vi "clusterParsing.vi"() -> ()   [LabVIEW 2009]
uses:
  Publisher/dataCluster.ctl
  <vilib>/vision/Image Controls.llb/IMAQ Image.ctl
panel:
  out "Array":string[](array[string])
  in  "Cluster in 2":T1
  in  "Data cluster StateM":T3
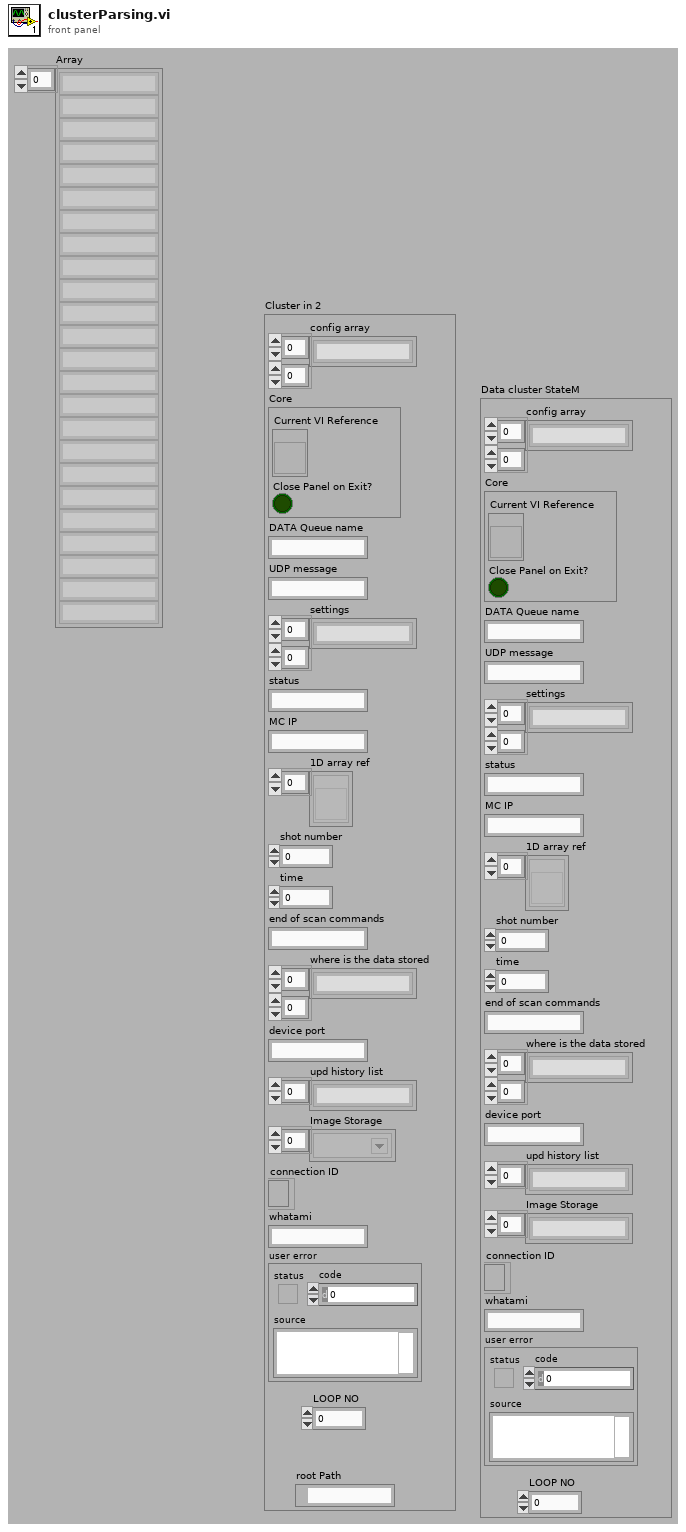
[diagram p1: front panel]
types:
  T1 = typedef "dataCluster.ctl" = cluster{"config array":string[][], "Core":cluster{"Current VI Reference":refnum<vi>, "Close Panel on Exit?":bool}, "DATA Queue name":string, "UDP message":string, "settings":string[][], "status":string, "MC IP":string, "1D array ref":refnum<vi>[], "shot number":i32, "time":u32, "end of scan commands":string, "where is the data stored":string[][], "device port":string, "upd history list":string[], "Image Storage":T2[], "connection ID":refnum<k16>, "whatami":string, "user error":errorcluster, "LOOP NO":u32, "root Path":path}
  T2 = typedef "IMAQ Image.ctl" = refnum<image>
  T3 = cluster{"config array":string[][], "Core":cluster{"Current VI Reference":refnum<vi>, "Close Panel on Exit?":bool}, "DATA Queue name":string, "UDP message":string, "settings":string[][], "status":string, "MC IP":string, "1D array ref":refnum<vi>[], "shot number":i32, "time":u32, "end of scan commands":string, "where is the data stored":string[][], "device port":string, "upd history list":string[], "Image Storage":string[], "connection ID":refnum<k16>, "whatami":string, "user error":errorcluster, "LOOP NO":u32}
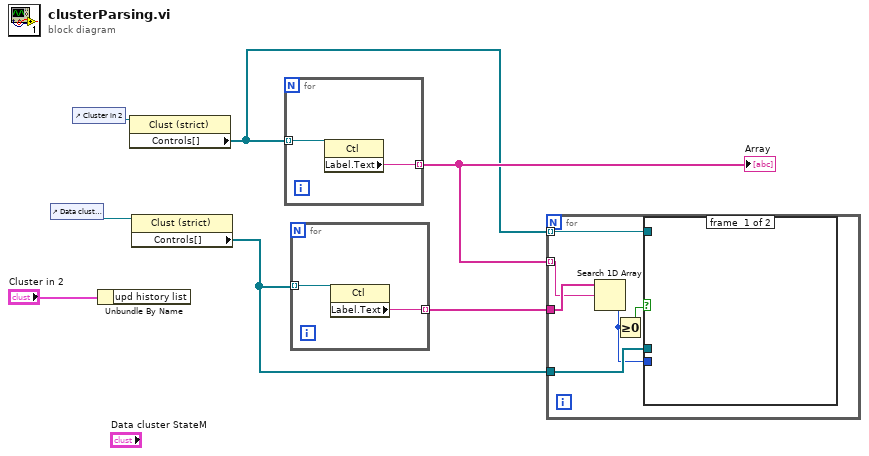
[diagram p0: block diagram]
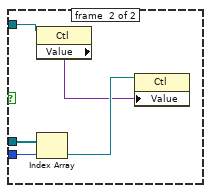
[diagram p2: hidden frame]
diagram:
  n1 = control-ref of="Data cluster StateM"() -> (w6:refnum<vi>)
  n2 = control-ref of="Cluster in 2"() -> (w7:refnum<vi>)
  n3 = Unbundle By Name("Cluster in 2") -> ()  [unwired: 1 out]
  n4 = property class="Clust (strict)"(reference=w7) -> ("Controls[]"=w2:refnum<vi>[])  [unwired: 1 in, 2 out]
  n5 = property class="Clust (strict)"(reference=w6) -> ("Controls[]"=w3:refnum<vi>[])  [unwired: 1 in, 2 out]
  n6 = for {
    tunnel: w2 -> [w9] mode=indexing
    tunnel: [w8] -> w5 mode=indexing
    n7 = property class="Ctl"(reference=w9) -> ("Label.Text"=w8:string)  [unwired: 1 in, 2 out]
  }
  "Array" <- w5
  n8 = for {
    tunnel: w3 -> [w11] mode=indexing
    tunnel: [w10] -> w4 mode=indexing
    n9 = property class="Ctl"(reference=w11) -> ("Label.Text"=w10:string)  [unwired: 1 in, 2 out]
  }
  n10 = for {
    tunnel: w5 -> [w16] mode=indexing
    tunnel: w4 -> [w17]
    tunnel: w3 -> [w15]
    tunnel: w2 -> [w14] mode=indexing
    n11 = Search 1D Array(1D array=w17, element=w16) -> (index of element=w13:i32)  [unwired: 1 in]
    n12 = Greater Or Equal To 0?(x=w13) -> (x >= 0?=w12:bool)
    n13 = case shown="True" w12 {
      tunnel: w15 -> [_ w22]
      tunnel: w13 -> [_ w21]
      tunnel: w14 -> [_ w19]
      frame #0 {
      }
      frame #1 {
        n14 = property class="Ctl"(reference=w19) -> ("Value"=w18:variant)  [unwired: 1 in, 2 out]
        n15 = Index Array(array=w22, index=w21) -> (element=w20:refnum<vi>)
        n16 = property class="Ctl"(reference=w20, "Value"=w18) -> ()  [unwired: 1 in, 2 out]
      }
    }
  }
